vi "休息提示.vi"(11 "Digital输入":refnum<vi>) -> ()   [LabVIEW 2016]
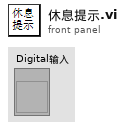
[diagram p1: front panel]
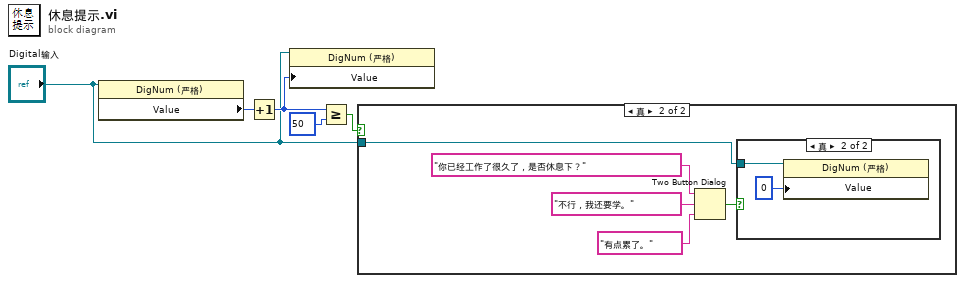
[diagram p0: block diagram]
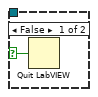
[diagram p3: hidden frame]
diagram:
  n1 = property class="DigNum (严格)"(reference="Digital输入") -> ("Value"=w4:i32)  [unwired: 1 in, 2 out]
  n2 = Increment(x=w4) -> (x+1=w5:i32)
  n3 = property class="DigNum (严格)"(reference="Digital输入", "Value"=w5) -> ()  [unwired: 1 in, 2 out]
  n4 = Greater Or Equal?(x=w5, y=50) -> (x >= y?=w3:bool)
  n5 = case shown="真" w3 {
    tunnel: "Digital输入" -> [_ w8]
    frame False {
    }
    frame True {
      n6 = Two Button Dialog(message="你已经工作了很久了，是否休息下？" ("消息"), 1:"有点累了。" ("T按钮名称（“确定”）"), 2:"不行，我还要学。" ("F按钮名称（“取消”）")) -> (T button?=w9:bool)
      n7 = case shown="真" w9 {
        selector: w9 -> [w11 _]
        tunnel: w8 -> [_ w12]
        frame False {
          n8 = Quit LabVIEW(quit? (T)=w11) -> ()
        }
        frame True {
          n9 = property class="DigNum (严格)"(reference=w12, "Value"=0 ("事件计数")) -> ()  [unwired: 1 in, 2 out]
        }
      }
    }
  }
